vi "Scale(Table).vi"(9 "coercion":T2, 10 "scales":T1[](array[typedef]), 11 "unscaled value":dbl format="%#_13g") -> (3 "scaled value":dbl)   [LabVIEW 2015, in "Scale.lvlib"]
uses:
  Scale.lvlib
  ScaleMapping.ctl
  Coercion.ctl
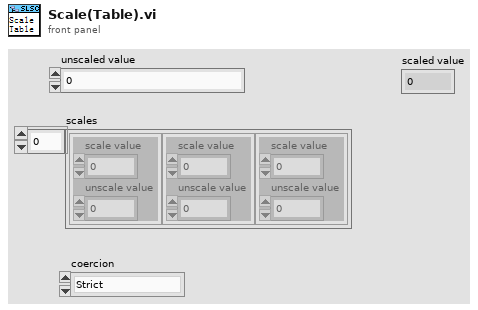
[diagram p1: front panel]
types:
  T1 = typedef "Scale.lvlib/ScaleMapping.ctl" = cluster{"scale value":dbl, "unscale value":dbl}
  T2 = typedef "Scale.lvlib/Coercion.ctl" = enum16{"Strict", "RoundToNearest", "Interpolate"}
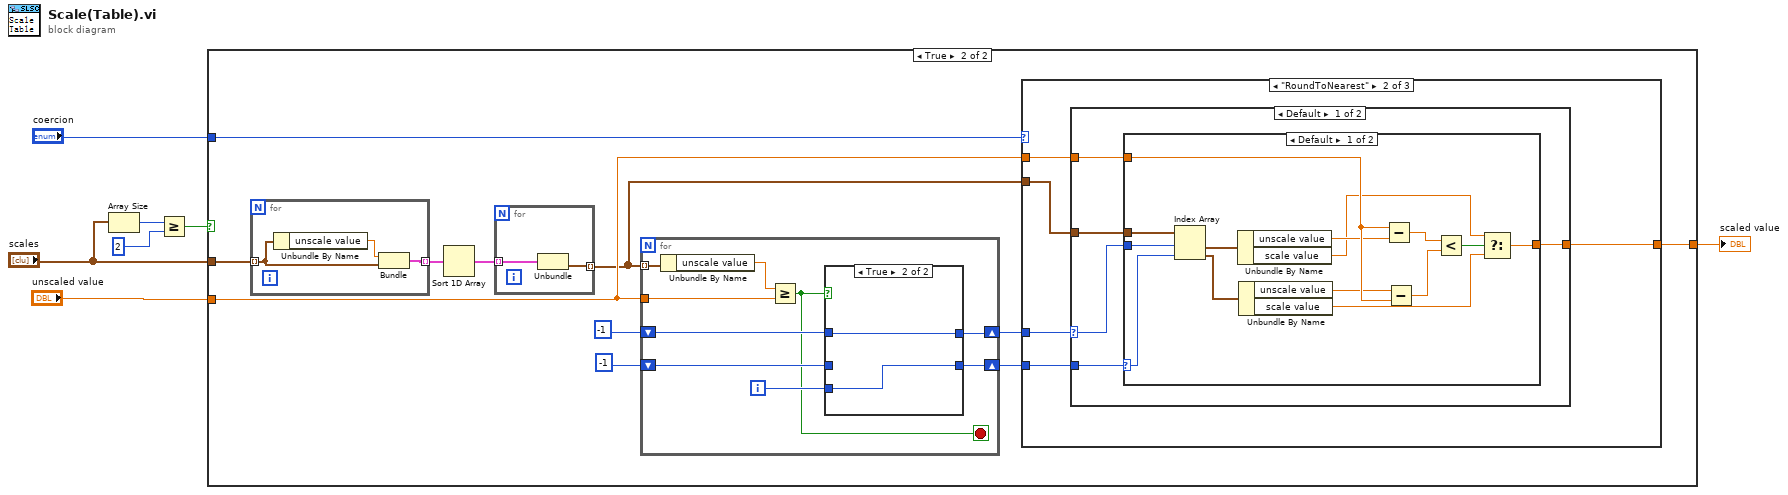
[diagram p0: block diagram]
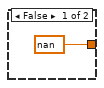
[diagram p2: hidden frame]
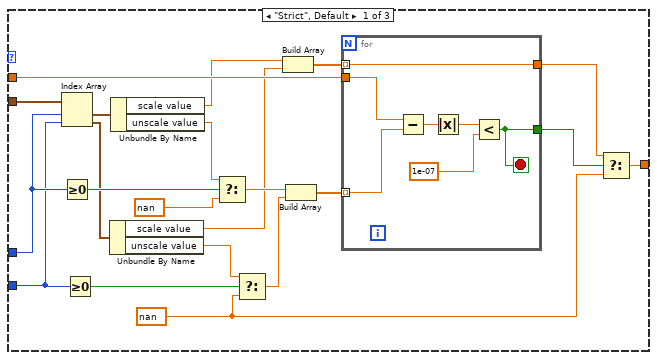
[diagram p3: hidden frame]
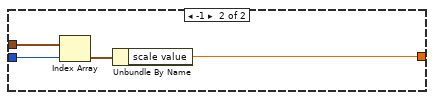
[diagram p4: hidden frame]
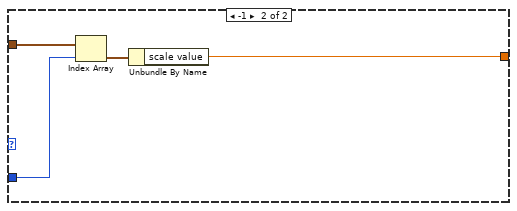
[diagram p5: hidden frame]
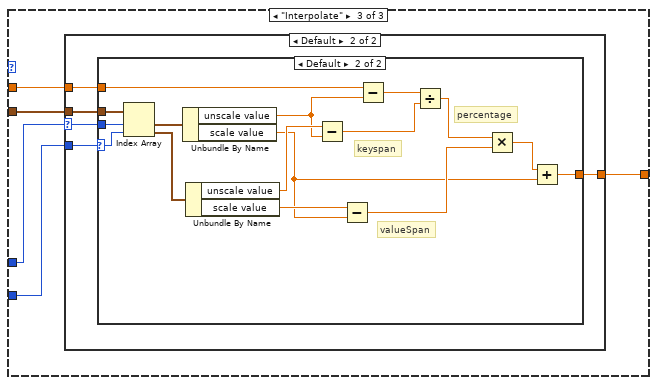
[diagram p6: hidden frame]
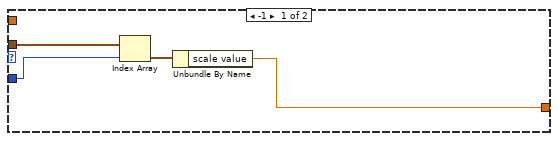
[diagram p7: hidden frame]
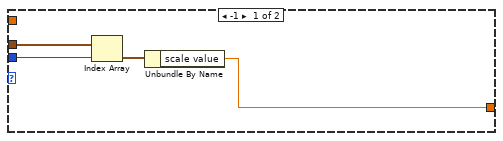
[diagram p8: hidden frame]
diagram:
  n1 = Array Size(array="scales") -> (size(s)=w5:i32)
  n2 = Greater Or Equal?(x=w5, y=2) -> (x >= y?=w4:bool)
  n3 = case shown="True" w4 {
    tunnel: "scales" -> [_ w12]
    tunnel: "coercion" -> [_ w17]
    tunnel: "unscaled value" -> [_ w14]
    tunnel: [nan ("f") w13] -> w6
    frame False {
    }
    frame True {
      n4 = for {
        tunnel: w12 -> [w24] mode=indexing
        tunnel: [w22] -> w11 mode=indexing
        n5 = Unbundle By Name(w24) -> ("unscale value"=w23:dbl)
        n6 = Bundle("unscale value"=w23, "scalue"=w24) -> (w22:cluster{"unscale value":dbl, "scalue":T1})  [unwired: 1 in]
      }
      n7 = Sort 1D Array(array=w11) -> (sorted array=w10:cluster{"unscale value":dbl, "scalue":T1}[])
      n8 = for {
        tunnel: w10 -> [w21] mode=indexing
        tunnel: [w20] -> w9 mode=indexing
        n9 = Unbundle(w21) -> ("scalue"=w20:T1)  [unwired: 1 out]
      }
      n10 = for {
        tunnel: w9 -> [w127] mode=indexing
        tunnel: w14 -> [w125]
        shift-right: [w122] -> w16
        shift-left: -1 -> [w121]
        shift-right: [w123] -> w15
        shift-left: -1 -> [w120]
        i -> [w124]
        stop <- w119 stop-if-true
        n11 = Unbundle By Name(w127) -> ("unscale value"=w126:dbl)
        n12 = Greater Or Equal?(x=w126, y=w125) -> (x >= y?=w119:bool)
        n13 = case shown="True" w119 {
          tunnel: w124 -> [w128 w131]
          tunnel: [w129 w131] -> w123
          tunnel: [w128 w130] -> w122
          tunnel: w121 -> [_ w130]
          tunnel: w120 -> [w129 _]
          frame False {
          }
          frame True {
          }
        }
      }
      n14 = case shown="\"RoundToNearest\"" w17 {
        tunnel: w16 -> [w44 w57 w85]
        tunnel: w15 -> [w41 w55 w88]
        tunnel: w9 -> [w30 w56 w89]
        tunnel: w14 -> [w33 w53 w87]
        tunnel: [w31 w54 w86] -> w13
        frame "Strict", Default {
          w25 = nan
          n15 = Index Array(array=w30, index #1=w44, index #2=w41) -> (element #1=w43:T1, element #2=w40:T1)
          n16 = Greater Or Equal To 0?(x=w44) -> (x >= 0?=w45:bool)
          n17 = Greater Or Equal To 0?(x=w41) -> (x >= 0?=w38:bool)
          n18 = Unbundle By Name(w40) -> ("scale value"=w26:dbl, "unscale value"=w39:dbl)
          n19 = Unbundle By Name(w43) -> ("scale value"=w27:dbl, "unscale value"=w42:dbl)
          n20 = Select(t=w42, s=w45, f=nan) -> (s? t:f=w36:dbl)
          n21 = Select(t=w39, s=w38, f=w25) -> (s? t:f=w35:dbl)
          n22 = Build Array(w27, w26) -> (w29:dbl[])
          n23 = Build Array(w36, w35) -> (w34:dbl[])
          n24 = for {
            tunnel: w34 -> [w51] mode=indexing
            tunnel: w33 -> [w52]
            tunnel: [w48] -> w32
            tunnel: w29 -> [w46] mode=indexing
            tunnel: [w46] -> w28
            stop <- w48 stop-if-true
            n25 = Subtract(x=w52, y=w51) -> (x-y=w50:dbl)
            n26 = Absolute Value(x=w50) -> (abs(x)=w47:dbl)
            n27 = Less?(x=w47, y=1e-07) -> (x < y?=w48:bool)
          }
          n28 = Select(t=w28, s=w32, f=w25) -> (s? t:f=w31:dbl)
        }
        frame "RoundToNearest" {
          n29 = case shown="Default" w57 {
            selector: w57 -> [w60 _]
            tunnel: w56 -> [w61 w81]
            tunnel: w55 -> [w62 w84]
            tunnel: [w59 w82] -> w54
            tunnel: w53 -> [w58 _]
            frame Default {
              n30 = case shown="Default" w62 {
                selector: w62 -> [w74 _]
                tunnel: w61 -> [w76 w79]
                tunnel: w60 -> [w75 w78]
                tunnel: [w66 w77] -> w59
                tunnel: w58 -> [w72 _]
                frame Default {
                  n31 = Index Array(array=w76, index #1=w75, index #2=w74) -> (element #1=w73:T1, element #2=w65:T1)
                  n32 = Unbundle By Name(w73) -> ("unscale value"=w68:dbl, "scale value"=w64:dbl)
                  n33 = Unbundle By Name(w65) -> ("unscale value"=w67:dbl, "scale value"=w63:dbl)
                  n34 = Subtract(x=w72, y=w68) -> (x-y=w71:dbl)
                  n35 = Subtract(x=w67, y=w72) -> (x-y=w70:dbl)
                  n36 = Less?(x=w71, y=w70) -> (x < y?=w69:bool)
                  n37 = Select(t=w64, s=w69, f=w63) -> (s? t:f=w66:dbl)
                }
                frame -1 {
                  n38 = Index Array(array=w79, index=w78) -> (element=w80:T1)
                  n39 = Unbundle By Name(w80) -> ("scale value"=w77:dbl)
                }
              }
            }
            frame -1 {
              n40 = Index Array(array=w81, index=w84) -> (element=w83:T1)
              n41 = Unbundle By Name(w83) -> ("scale value"=w82:dbl)
            }
          }
        }
        frame "Interpolate" {
          n42 = case shown="Default" w85 {
            selector: w85 -> [_ w95]
            tunnel: w89 -> [w93 w98]
            tunnel: w88 -> [w92 w94]
            tunnel: w87 -> [_ w97]
            tunnel: [w90 w96] -> w86
            frame -1 {
              n43 = Index Array(array=w93, index=w92) -> (element=w91:T1)
              n44 = Unbundle By Name(w91) -> ("scale value"=w90:dbl)
            }
            frame Default {
              n45 = case shown="Default" w94 {
                selector: w94 -> [_ w107]
                tunnel: w98 -> [w101 w118]
                tunnel: w97 -> [_ w116]
                tunnel: [w99 w110] -> w96
                tunnel: w95 -> [w100 w109]
                frame -1 {
                  n46 = Index Array(array=w101, index=w100) -> (element=w102:T1)
                  n47 = Unbundle By Name(w102) -> ("scale value"=w99:dbl)
                }
                frame Default {
                  # "percentage"
                  # "keyspan"
                  # "valueSpan"
                  n48 = Index Array(array=w118, index #1=w109, index #2=w107) -> (element #1=w117:T1, element #2=w108:T1)
                  n49 = Unbundle By Name(w117) -> ("unscale value"=w105:dbl, "scale value"=w103:dbl)
                  n50 = Unbundle By Name(w108) -> ("unscale value"=w106:dbl, "scale value"=w104:dbl)
                  n51 = Subtract(x=w106, y=w105) -> (x-y=w112:dbl)
                  n52 = Subtract(x=w104, y=w103) -> (x-y=w113:dbl)
                  n53 = Subtract(x=w116, y=w105) -> (x-y=w115:dbl)
                  n54 = Divide(x=w115, y=w112) -> (x/y=w114:dbl)
                  n55 = Multiply(x=w114, y=w113) -> (x*y=w111:dbl)
                  n56 = Add(x=w111, y=w103) -> (x+y=w110:dbl)
                }
              }
            }
          }
        }
      }
    }
  }
  "scaled value" <- w6
